vi "Update Input Polarity.vi"   [LabVIEW 2014, in "MCP23S17.lvlib"]
doc: "Sets the input polarity of the pins on the chip."
uses:
  MCP23S17.lvlib
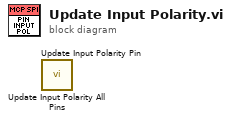
[diagram p0: block diagram]
diagram:
  n1 = call "Update Input Polarity All Pins.vi"() -> ()  [unwired: 9 in, 3 out]
  n2 = call "Update Input Polarity Pin.vi"() -> ()  [unwired: 9 in, 3 out]
